vi "p2.vi"() -> ()   [LabVIEW 2023, in "d24.lvlib"]
uses:
  d24.lvlib
  AOC/AOC.lvlib
  <vilib>/Analysis/NI_AALPro.lvlib
  <vilib>/Analysis/7linalg.llb/Solve Linear Equations (single right hand).vi
panel:
  out "Rock":T1={"x"=10, "y"=10, "z"=10, "vx"=10, "vy"=10, "vz"=10}
  in  "Example":string="19, 13, 30 @ -2,  1, -2\n18, 19, 22 @ -1, -1, -2\n20, 25, 34 @ -2, -2, -4\n12, 31, 28 @ -1, -2, -1\n20, 19, 15 @  1, -5, -3"
  in  "Example":bool=TRUE
  out "Answer":i64=10
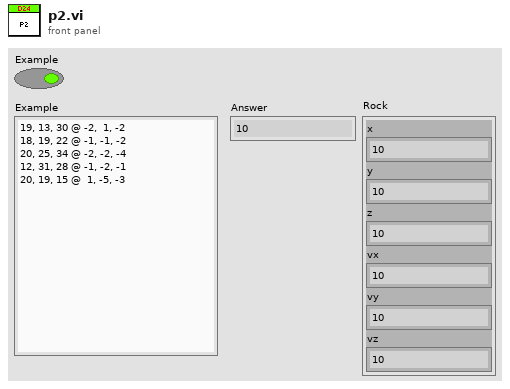
[diagram p1: front panel]
types:
  T1 = cluster{"x":i64, "y":i64, "z":i64, "vx":i64, "vy":i64, "vz":i64}
  T2 = cluster{"X[0]":ext, "X[1]":ext, "X[2]":ext, "X[3]":ext, "X[4]":ext, "X[5]":ext}
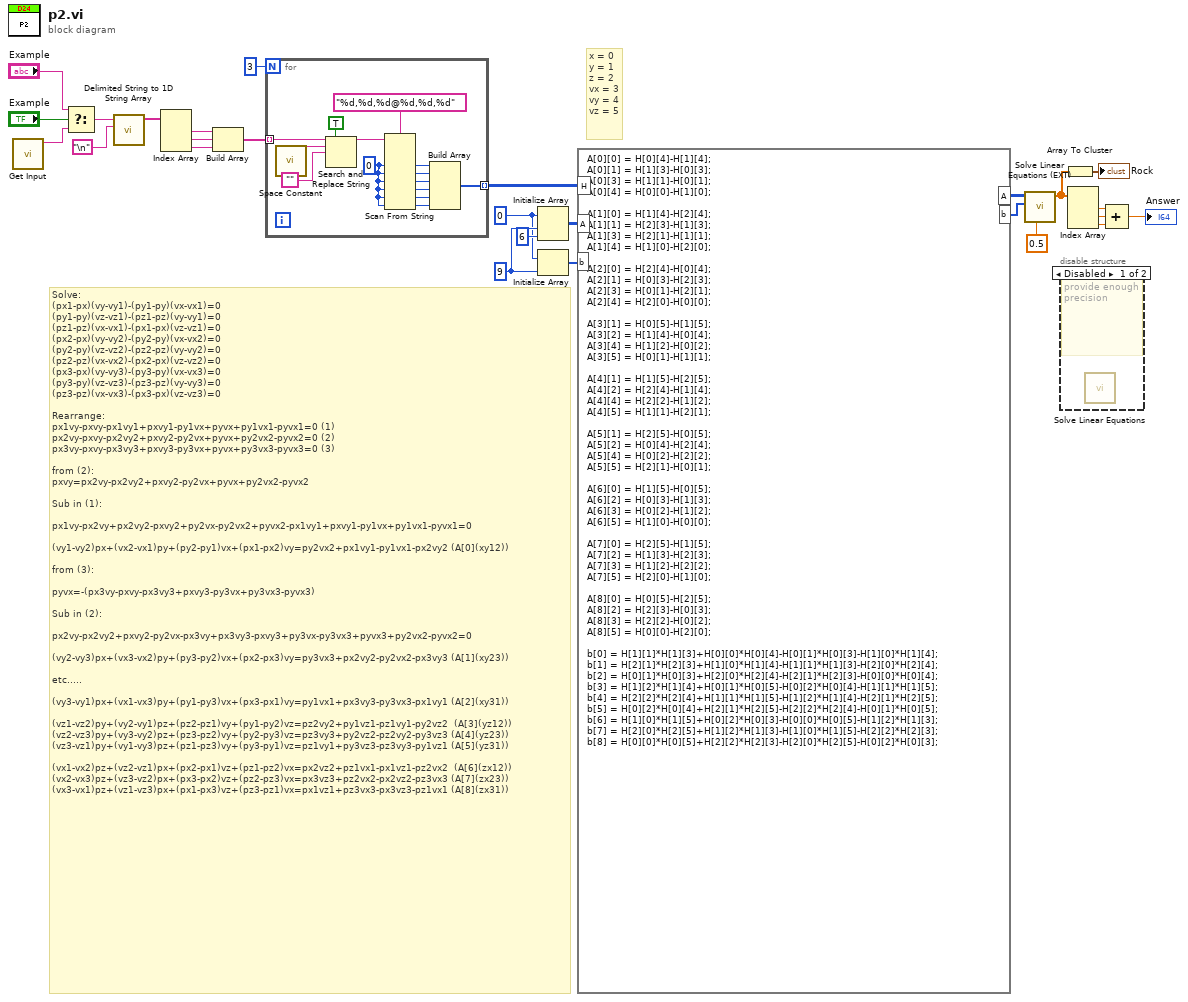
[diagram p0: block diagram]
diagram:
  w8 = 9 ("dimension size")
  w7 = i64 0 ("default value 1")
  # "x = 0\ny = 1\nz = 2\nvx = 3\nvy = 4\nvz = 5"
  # "Solve:\n(px1-px)(vy-vy1)-(py1-py)(vx-vx1)=0\n(py1-py)(vz-vz1)-(pz1-pz)(vy-vy1)=0\n(pz1-pz)(vx-vx1)-(px1-px)(vz-vz1)=0\n(px2-px)(vy-vy2)-(py2-py)(vx-vx2)=0\n(py2-py)(vz-vz2)-(pz2-pz)(vy-vy2)=0\n(pz2-pz)(vx-vx2)-(px2-px)(vz-vz2)=0\n(px3-px)(vy-vy3)-(py3-py)(vx-vx3)=0\n(py3-py)(vz-vz3)-(pz3-pz)(vy-vy3)=0\n(pz3-pz)(vx-vx3)-(px3-px)(vz-vz3)=0\n\nRearrange:\npx1vy-pxvy-px1vy1+pxvy1-py1vx+pyvx+py1vx1-pyvx1=0 (1)\npx2vy-pxvy-px2vy2+pxvy2-py2vx+pyvx+py2vx2-pyvx2=0 (2)\npx3vy-pxvy-px3vy3+pxvy3-py3vx+pyvx+py3vx3-pyvx3=0 (3)\n\nfrom (2):\npxvy=px2vy-px2vy2+pxvy2-py2vx+pyvx+py2vx2-pyvx2\n\nSub in (1):\n\npx1vy-px2vy+px2vy2-pxvy2+py2vx-py2vx2+pyvx2-px1vy1+pxvy1-py1vx+py1vx1-pyvx1=0\n\n(vy1-vy2)px+(vx2-vx1)py+(py2-py1)vx+(px1-px2)vy=py2vx2+px1vy1-py1vx1-px2vy2 (A[0](xy12))\n\nfrom (3):\n\npyvx=-(px3vy-pxvy-px3vy3+pxvy3-py3vx+py3vx3-pyvx3)\n\nSub in (2):\n\npx2vy-px2vy2+pxvy2-py2vx-px3vy+px3vy3-pxvy3+py3vx-py3vx3+pyvx3+py2vx2-pyvx2=0\n\n(vy2-vy3)px+(vx3-vx2)py+(py3-py2)vx+(px2-px3)vy=py3vx3+px2vy2-py2vx2-px3vy3 (A[1](xy23))\n\netc.....\n\n(vy3-vy1)px+(vx1-vx3)py+(py1-py3)vx+(px3-px1)vy=py1vx1+px3vy3-py3vx3-px1vy1 (A[2](xy31))\n\n(vz1-vz2)py+(vy2-vy1)pz+(pz2-pz1)vy+(py1-py2)vz=pz2vy2+py1vz1-pz1vy1-py2vz2  (A[3](yz12))\n(vz2-vz3)py+(vy3-vy2)pz+(pz3-pz2)vy+(py2-py3)vz=pz3vy3+py2vz2-pz2vy2-py3vz3 (A[4](yz23))\n(vz3-vz1)py+(vy1-vy3)pz+(pz1-pz3)vy+(py3-py1)vz=pz1vy1+py3vz3-pz3vy3-py1vz1 (A[5](yz31))\n\n(vx1-vx2)pz+(vz2-vz1)px+(px2-px1)vz+(pz1-pz2)vx=px2vz2+pz1vx1-px1vz1-pz2vx2  (A[6](zx12))\n(vx2-vx3)pz+(vz3-vz2)px+(px3-px2)vz+(pz2-pz3)vx=px3vz3+pz2vx2-px2vz2-pz3vx3 (A[7](zx23))\n(vx3-vx1)pz+(vz1-vz3)px+(px1-px3)vz+(pz3-pz1)vx=px1vz1+pz3vx3-px3vz3-pz1vx1 (A[8](zx31))"
  n1 = call "Get Input.vi"() -> ("Input"=w26:string)  [unwired: 11 in]
  n2 = Select(t="Example", s="Example", f=w26) -> (s? t:f=w24:string)
  n3 = call <vilib>:"Delimited String to 1D String Array.vi"("delimiter"="\n", "delimited string"=w24) -> ("string array"=w21:string[])  [unwired: 9 in]
  n4 = Index Array(array=w21) -> (element #1=w20:string, element #2=w18:string, element #3=w17:string)  [unwired: 3 in]
  n5 = Build Array(w20, w18, w17) -> (w19:string[])
  n6 = for {
    N: 3 -> [_]
    tunnel: w19 -> [w38] mode=indexing
    tunnel: [w27] -> w11 mode=indexing
    w34 = i64 0 ("default value 1")
    n7 = call <vilib>:"Space Constant.vi"() -> ("String"=w37:string)
    n8 = Search and Replace String(replace all?=TRUE ("replace all? (F)"), input string=w38, search string=w37, replace string="") -> (result string=w39:string)  [unwired: 4 in, 3 out]
    n9 = Scan From String(format string="%d,%d,%d@%d,%d,%d", input string=w39, default 1=w34, default 2=w34, default 3=w34, default 4=w34, default 5=w34, default 6=w34) -> (output 1=w33:i64, output 2=w32:i64, output 3=w31:i64, output 4=w30:i64, output 5=w29:i64, output 6=w28:i64)  [unwired: 2 in, 3 out]
    n10 = Build Array(w33, w32, w31, w30, w29, w28) -> (w27:i64[])
  }
  n11 = Initialize Array(w7, w8, 6 ("dimension size")) -> (w9:i64[][])
  n12 = Initialize Array(w7, w8) -> (w6:i64[])
  n13 = formula code="A[0][0] = H[0][4]-H[1][4];\nA[0][1] = H[1][3]-H[0][3];\nA[0][3] = H[1][1]-H[0][1];\nA[0][4] = H[0][0]-H[1][0];\n\nA[1][0] = H[1][4]-H[2][4];\nA[1][1] = H[2][3]-H[1][3];\nA[1][3] = H[2][1]-H[1][1];\nA[1][4] = H[1][0]-H[2][0];\n\nA[2][0] = H[2][4]-H[0][4];\nA[2][1] = H[0][3]-H[2][3];\nA[2][3] = H[0][1]-H[2][1];\nA[2][4] = H[2][0]-H[0][0];\n\nA[3][1] = H[0][5]-H[1][5];\nA[3][2] = H[1][4]-H[0][4];\nA[3][4] = H[1][2]-H[0][2];\nA[3][5] = H[0][1]-H[1][1];\n\nA[4][1] = H[1][5]-H[2][5];\nA[4][2] = H[2][4]-H[1][4];\nA[4][4] = H[2][2]-H[1][2];\nA[4][5] = H[1][1]-H[2][1];\n\nA[5][1] = H[2][5]-H[0][5];\nA[5][2] = H[0][4]-H[2][4];\nA[5][4] = H[0][2]-H[2][2];\nA[5][5] = H[2][1]-H[0][1];\n\nA[6][0] = H[1][5]-H[0][5];\nA[6][2] = H[0][3]-H[1][3];\nA[6][3] = H[0][2]-H[1][2];\nA[6][5] = H[1][0]-H[0][0];\n\nA[7][0] = H[2][5]-H[1][5];\nA[7][2] = H[1][3]-H[2][3];\nA[7][3] = H[1][2]-H[2][2];\nA[7][5] = H[2][0]-H[1][0];\n\nA[8][0] = H[0][5]-H[2][5];\nA[8][2] = H[2][3]-H[0][3];\nA[8][3] = H[2][2]-H[0][2];\nA[8][5] = H[0][0]-H[2][0];\n\nb[0] = H[1][1]*H[1][3]+H[0][0]*H[0][4]-H[0][1]*H[0][3]-H[1][0]*H[1][4];\nb[1] = H[2][1]*H[2][3]+H[1][0]*H[1][4]-H[1][1]*H[1][3]-H[2][0]*H[2][4];\nb[2] = H[0][1]*H[0][3]+H[2][0]*H[2][4]-H[2][1]*H[2][3]-H[0][0]*H[0][4];\nb[3] = H[1][2]*H[1][4]+H[0][1]*H[0][5]-H[0][2]*H[0][4]-H[1][1]*H[1][5];\nb[4] = H[2][2]*H[2][4]+H[1][1]*H[1][5]-H[1][2]*H[1][4]-H[2][1]*H[2][5];\nb[5] = H[0][2]*H[0][4]+H[2][1]*H[2][5]-H[2][2]*H[2][4]-H[0][1]*H[0][5];\nb[6] = H[1][0]*H[1][5]+H[0][2]*H[0][3]-H[0][0]*H[0][5]-H[1][2]*H[1][3];\nb[7] = H[2][0]*H[2][5]+H[1][2]*H[1][3]-H[1][0]*H[1][5]-H[2][2]*H[2][3];\nb[8] = H[0][0]*H[0][5]+H[2][2]*H[2][3]-H[2][0]*H[2][5]-H[0][2]*H[0][3];"("H"=w11, "A"=w9, "b"=w6) -> ("A"=w5:i64[][], "b"=w4:i64[])
  n14 = call "Solve Linear Equations (EXT).vi"("Tolerance"=0.5, "b"=w4, "A"=w5) -> ("X"=w2:ext[])  [unwired: 8 in]
  n15 = disable-structure shown="Disabled" {
    frame Disabled {
      # "This does not provide enough precision"
      n16 = call-poly <vilib>:"Solve Linear Equations.vi"() -> ()  [unwired: 3 in, 2 out]
    }
    frame Enabled {
    }
  }
  n17 = Array To Cluster(array=w2) -> (cluster=→"Rock":T2)
  n18 = Index Array(array=w2) -> (element #1=w15:ext, element #2=w14:ext, element #3=w13:ext)  [unwired: 3 in]
  n19 = Compound Arithmetic op=ADD(w15, w14, w13) -> (→"Answer":ext)
